vi "test_Add Array Type Cast .vi"(8 "error in (no error)":errorcluster, 11 "TestCase in":refnum<class "Instrument Addon Scripting API Channels Unit Tests.lvclass">) -> (0 "error out":errorcluster, 3 "TestCase out":refnum<class "Instrument Addon Scripting API Channels Unit Tests.lvclass">)   [LabVIEW 2018, in "Instrument Addon Scripting API Channels Unit Tests.lvclass"]
uses:
  Instrument Addon Scripting API Channels Unit Tests.lvclass
  APIs/Scripting API/TypeDefs/Array Type Cast Settings.ctl
  APIs/Scripting API/TypeDefs/Array Element.ctl
  Addon/Addon Shared/Types/Type Cast Type.ctl
  Addon/Addon Shared/Types/Endian.ctl
  Instrument Addon Scripting API Channels Unit Tests.lvclass/Instrument Addon Scripting API Channels Unit Tests.ctl
  Addon/Addon Shared/SubVIs/Constants.vi
  <vilib>/NI/NI VeriStand Advanced SysDef API/_SubVIs/SysDef.Search.GUID.vi
  <vilib>/NI/NI VeriStand Advanced SysDef API/_SubVIs/SysDef.Search.GUIDs.vi
  APIs/Scripting API/Channels/Create Data Channel - Array - Type Cast.vi
  <vilib>/NI Veristand/Custom Device API/Get Item Property (String).vi
  <vilib>/NI Veristand/Custom Device API/Get Item Property (U16).vi
  <vilib>/addons/_JKI Toolkits/VI Tester/TestCase.llb/TestCase.lvclass
  Instrument Addon Scripting API Test Assets/Instrument Addon Scripting API Test Assets.lvclass
  <vilib>/NI/NI VeriStand Advanced SysDef API/SysDef API/Advanced System Definition.lvlib
  Addon/Addon Shared/Instrument Addon Shared.lvlib
  APIs/Scripting API/Instrument Addon Scripting API.lvlib
  <vilib>/NI Veristand/Custom Device API/Custom Device API.lvlib
  C:/Program Files (x86)/National Instruments/LabVIEW 2018/vi.lib/addons/_JKI Toolkits/VI Tester/TestCase.llb/TestCase.lvclass
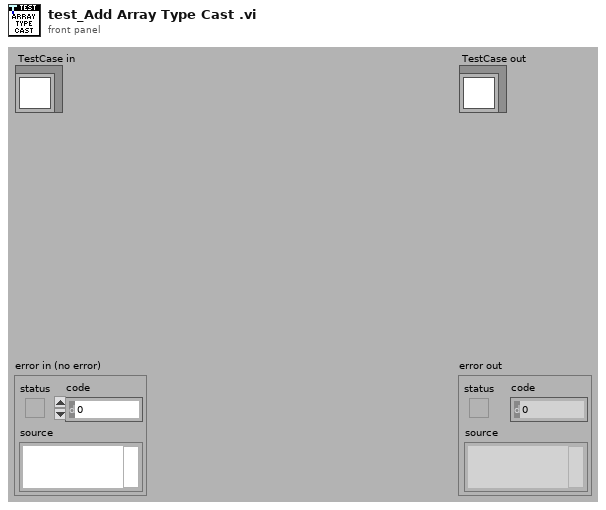
[diagram p1: front panel]
types:
  T1 = typedef "Instrument Addon Scripting API.lvlib/Array Type Cast Settings.ctl" = cluster{"Elements":T2[], "Type":T3, "Endian":T4, "Delimiter":string}
  T2 = typedef "Instrument Addon Scripting API.lvlib/Array Element.ctl" = cluster{"Name":string, "Default Value":dbl, "Units":string}
  T3 = typedef "Instrument Addon Shared.lvlib/Type Cast Type.ctl" = enum16{"DBL", "SGL", "U64", "U32", "U16", "U8", "I64", "I32", "I16", "I8"}
  T4 = typedef "Instrument Addon Shared.lvlib/Endian.ctl" = enum16{"Native", "Little", "Big"}
  T5 = typedef "Custom Device API.lvlib/Custom Device Item Ref.ctl" = u64
  T6 = typedef "Advanced System Definition.lvlib/TreeItem.Info.ctl" = cluster{"Name":string, "Description":string, "GUID":string, "Is Channel":bool, "Channel":T7, "Is Waveform":bool, "Waveform":T9}
  T7 = typedef "Custom Device API.lvlib/Custom Device Channel.ctl" = cluster{"Type":T8, "Units":string, "Default Value":dbl, "Faultable":bool, "Scalable":bool}
  T8 = typedef "Custom Device API.lvlib/Custom Device Channel Type.ctl" = enum16{"Input", "Output"}
  T9 = typedef "Custom Device API.lvlib/Custom Device Waveform.ctl" = cluster{"Data Type":T10, "Units":string}
  T10 = typedef "Custom Device API.lvlib/Custom Device Waveform DataType.ctl" = enum16{"Double", "Complex Double"}
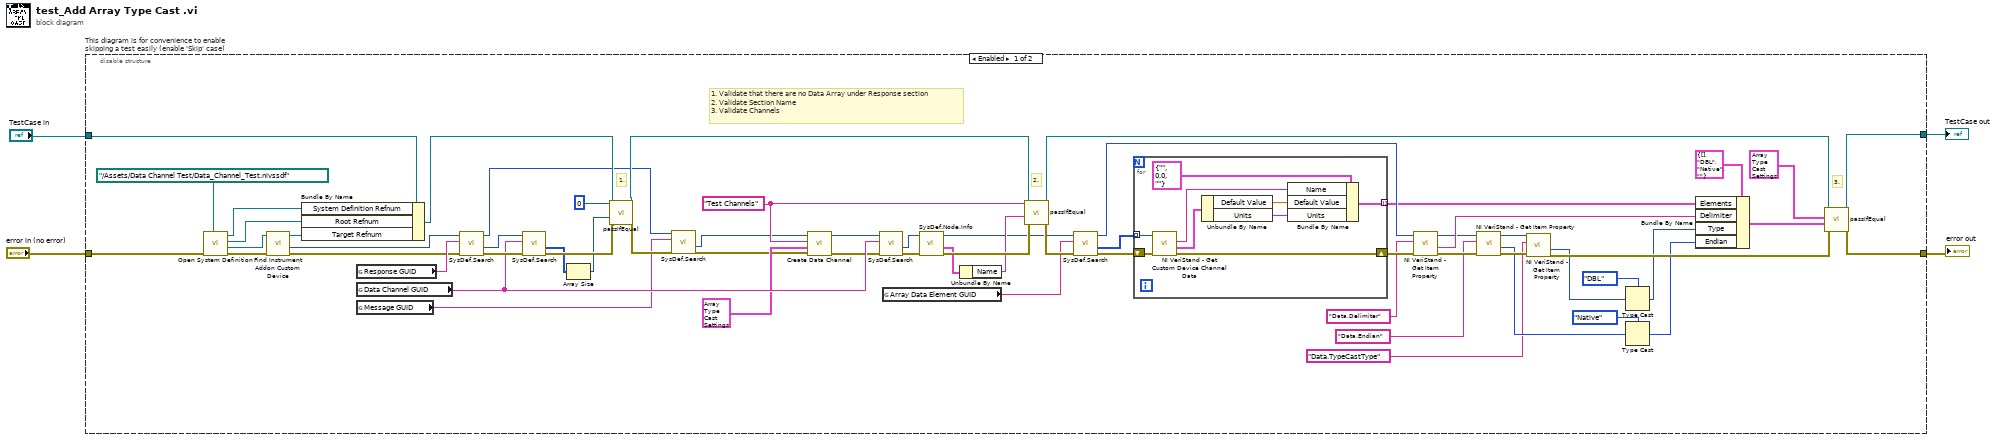
[diagram p0: block diagram]
diagram:
  n1 = disable-structure "This diagram is for convenience to enable skipping a test easily (enable 'Skip' case)" shown="Enabled" {
    disable-tunnel: "TestCase in" -> [w16 w80]
    disable-tunnel: [w39 w78] -> w1
    disable-tunnel: [w40 w79] -> w3
    disable-tunnel: "error in (no error)" -> [w64 w77]
    frame Enabled {
      w53 = "Test Channels" ("Name")
      # "3."
      # "2."
      # "1. Validate that there are no Data Array under Response section\n2. Validate Section Name\n3. Validate Channels"
      # "1."
      n2 = call "Open System Definition.vi"("error in (no error)"=w64, "System Definition File"=path "../Assets/Data Channel Test/Data_Channel_Test.nivssdf") -> ("error out"=w67:errorcluster, "Target Refnum"=w66:refnum<k24>, "Root Refnum"=w14:refnum<k24>, "System Definition Refnum"=w15:refnum<k24>)  [unwired: 6 in]
      n3 = call "Find Instrument Addon Custom Device.vi"("error in"=w67, "target in"=w66) -> ("error out"=w17:errorcluster, "NodeID"=w63:u64, "target out"=w13:refnum<k24>)  [unwired: 7 in]
      n4 = Bundle By Name(cluster=w16, "System Definition Refnum"=w15, "Root Refnum"=w14, "Target Refnum"=w13) -> (w12:refnum<class "Instrument Addon Scripting API Channels Unit Tests.lvclass">)
      n5 = global read "Constants.vi" "Response GUID"() -> (w62:string)
      n6 = global read "Constants.vi" "Data Channel GUID"() -> (w59:string)
      n7 = global read "Constants.vi" "Message GUID"() -> (w8:string)
      n8 = call-poly <vilib>:"SysDef.Search.vi"("error in (no error)"=w17, "GUID"=w62, "nodeID"=w63) -> ("error out"=w60:errorcluster, "Value out"=w61:u64, "nodeID out"=w7:u64)  [unwired: 5 in, 1 out]
      n9 = call-poly <vilib>:"SysDef.Search.vi"("error in (no error)"=w60, "GUID"=w59, "nodeID"=w61) -> ("error out"=w57:errorcluster, "Values Out"=w56:u64[])  [unwired: 5 in, 2 out]
      n10 = Array Size(array=w56) -> (size(s)=w55:i32)
      n11 = call-dynamic "passIfEqual.vi"("error in (no error)"=w57, "y"=w55, "x"=0 ("size(s)"), "TestCase in"=w12) -> ("error out"=w11:errorcluster, "TestCase out"=w58:refnum<class "Instrument Addon Scripting API Channels Unit Tests.lvclass">)  [unwired: 6 in]
      n12 = call-poly <vilib>:"SysDef.Search.vi"("error in (no error)"=w11, "GUID"=w8, "nodeID"=w7) -> ("error out"=w10:errorcluster, "Value out"=w9:u64)  [unwired: 5 in, 2 out]
      n13 = call-poly "Create Data Channel.vi"("Error In"=w10, "Settings"=T1 {"Elements"=[{"Name"="Wait Time", "Default Value"=2.0, "Units"="ms"}, {"Name"="Rate", "Default Value"=15.0, "Units"="Hz"}], "Type"=enum."I8", "Endian"=enum."Little", "Delimiter"="_"}, "Name"=w53, "Message Refnum In"=w9) -> ("Error Out"=w52:errorcluster, "Message Refnum Out"=w51:T5)  [unwired: 5 in, 1 out]
      n14 = call-poly <vilib>:"SysDef.Search.vi"("error in (no error)"=w52, "GUID"=w59, "nodeID"=w51) -> ("error out"=w50:errorcluster, "Value out"=w49:u64)  [unwired: 5 in, 2 out]
      n15 = global read "Constants.vi" "Array Data Element GUID"() -> (w42:string)
      n16 = call <vilib>:"SysDef.Node.Info.vi"("error in (no error)"=w50, "nodeID"=w49) -> ("error out"=w48:errorcluster, "Item Info"=w47:T6, "nodeID out"=w43:u64)  [unwired: 6 in, 1 out]
      n17 = Unbundle By Name(w47) -> ("Name"=w46:string)
      n18 = call-dynamic "passIfEqual.vi"("error in (no error)"=w48, "y"=w46, "x"=w53, "TestCase in"=w58) -> ("error out"=w45:errorcluster, "TestCase out"=w34:refnum<class "Instrument Addon Scripting API Channels Unit Tests.lvclass">)  [unwired: 6 in]
      n19 = call-poly <vilib>:"SysDef.Search.vi"("error in (no error)"=w45, "GUID"=w42, "nodeID"=w43) -> ("error out"=w44:errorcluster, "Values Out"=w41:u64[], "nodeID out"=w37:u64)  [unwired: 5 in, 1 out]
      n20 = for {
        shift-right: [w68] -> w38
        shift-left: w44 -> [w75]
        tunnel: w41 -> [w76] mode=indexing
        tunnel: [w69] -> w36 mode=indexing
        n21 = call <vilib>:"NI VeriStand - Get Custom Device Channel Data.vi"("error in (no error)"=w75, "Channel Ref in"=w76) -> ("error out"=w68:errorcluster, "Channel"=w72:T7, "Channel Name"=w73:string)  [unwired: 4 in, 3 out]
        n22 = Unbundle By Name(w72) -> ("Default Value"=w70:dbl, "Units"=w71:string)
        n23 = Bundle By Name(cluster=T2 {"Name"="", "Default Value"=0.0, "Units"=""} ("Array Element"), "Name"=w73, "Default Value"=w70, "Units"=w71) -> (w69:T2)
      }
      n24 = call-poly <vilib>:"NI VeriStand - Get Item Property.vi"("error in (no error)"=w38, "Property Name"="Data.Delimiter", "Item Ref in"=w37) -> ("error out"=w28:errorcluster, "Value"=w31:string, "Item Ref out"=w26:T5)  [unwired: 5 in, 1 out]
      n25 = call-poly <vilib>:"NI VeriStand - Get Item Property.vi"("error in (no error)"=w28, "Property Name"="Data.Endian", "Item Ref in"=w26) -> ("error out"=w27:errorcluster, "Value"=w24:u16, "Item Ref out"=w25:T5)  [unwired: 5 in, 1 out]
      n26 = call-poly <vilib>:"NI VeriStand - Get Item Property.vi"("error in (no error)"=w27, "Property Name"="Data.TypeCastType", "Item Ref in"=w25) -> ("error out"=w35:errorcluster, "Value"=w30:u16)  [unwired: 5 in, 2 out]
      n27 = Type Cast(type=Type_Cast_Type."DBL" ("Type"), x=w30) -> (*(type *) &x=w29:T3)
      n28 = Type Cast(type=Endian."Native" ("Endian"), x=w24) -> (*(type *) &x=w23:T4)
      n29 = Bundle By Name(cluster=T1 {"Elements"=[], "Type"=enum."DBL", "Endian"=enum."Native", "Delimiter"=""} ("Settings"), "Elements"=w36, "Delimiter"=w31, "Type"=w29, "Endian"=w23) -> (w6:T1)
      n30 = call-dynamic "passIfEqual.vi"("error in (no error)"=w35, "y"=w6, "x"=T1 {"Elements"=[{"Name"="Wait Time", "Default Value"=2.0, "Units"="ms"}, {"Name"="Rate", "Default Value"=15.0, "Units"="Hz"}], "Type"=enum."I8", "Endian"=enum."Little", "Delimiter"="_"} ("Settings"), "TestCase in"=w34) -> ("error out"=w40:errorcluster, "TestCase out"=w39:refnum<class "Instrument Addon Scripting API Channels Unit Tests.lvclass">)  [unwired: 6 in]
    }
    frame Disabled {
      # "skip test result while test is under development"
      n31 = call <vilib>:"skip.vi"("error in (no error)"=w77, "TestCase in"=w80) -> ("error out"=w79:errorcluster, "TestCase out"=w78:refnum<class "Instrument Addon Scripting API Channels Unit Tests.lvclass">)  [unwired: 8 in]
    }
  }
  "error out" <- w3
  "TestCase out" <- w1
